vi "differentiator.vi"(10 "X-YCluster":cluster{"Array":dbl[], "Array":dbl[]}) -> (1 "sign":dbl[](array[numeric]), 2 "deltaY/deltaX":dbl[](array[numeric]) format="%#.2f")   [LabVIEW 2022 SP3]
panel:
  out "Ys":dbl[](array[numeric])
  out "Xs":dbl[](array[numeric]) format="%#.2f"
  # "Computes gradient using central difference method; also reports sign of gradient."
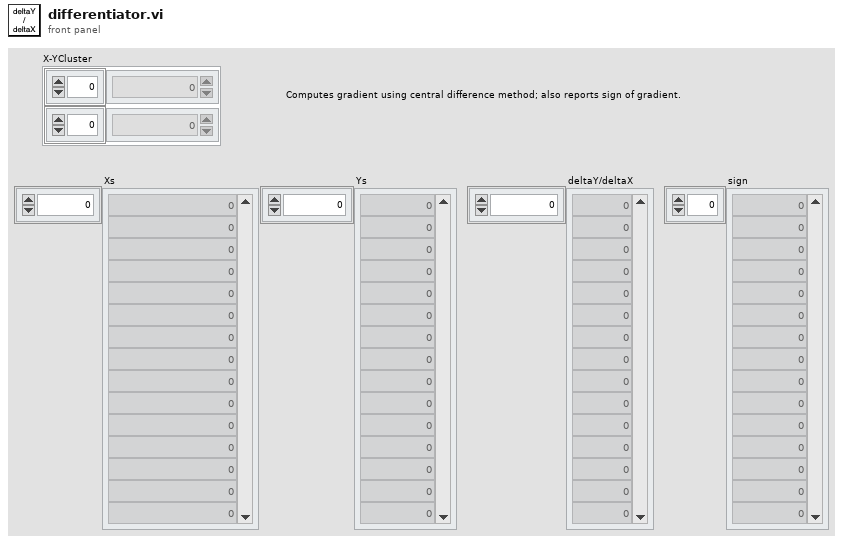
[diagram p1: front panel]
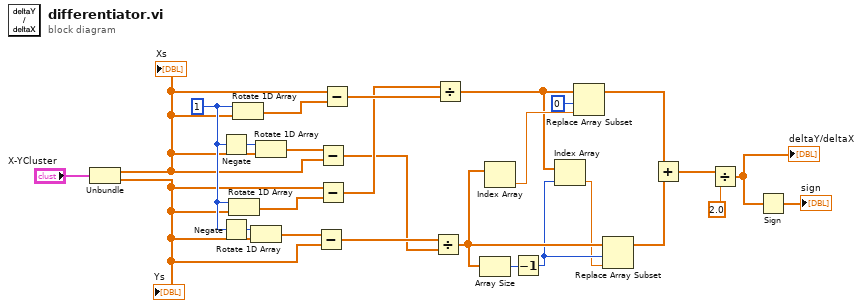
[diagram p0: block diagram]
diagram:
  w20 = 1 ("n")
  n1 = Unbundle("X-YCluster") -> ("Array"=w14:dbl[], "Array"=w17:dbl[])
  "Xs" <- w14
  "Ys" <- w17
  n2 = Negate(x=w20) -> (-x=w19:i32)
  n3 = Negate(x=w20) -> (-x=w21:i32)
  n4 = Rotate 1D Array(1:w17, 2:w20) -> (0:w25:dbl[])
  n5 = Rotate 1D Array(1:w14, 2:w20) -> (0:w26:dbl[])
  n6 = Rotate 1D Array(1:w17, 2:w21) -> (0:w18:dbl[])
  n7 = Rotate 1D Array(1:w14, 2:w19) -> (0:w15:dbl[])
  n8 = Subtract(x=w18, y=w17) -> (x-y=w13:dbl[])
  n9 = Subtract(x=w15, y=w14) -> (x-y=w12:dbl[])
  n10 = Subtract(x=w17, y=w25) -> (x-y=w16:dbl[])
  n11 = Subtract(x=w14, y=w26) -> (x-y=w24:dbl[])
  n12 = Divide(x=w13, y=w12) -> (x/y=w5:dbl[])
  n13 = Divide(x=w16, y=w24) -> (x/y=w3:dbl[])
  n14 = Array Size(array=w5) -> (size(s)=w11:i32)
  n15 = Index Array(array=w5) -> (element=w4:dbl)  [unwired: 1 in]
  n16 = Decrement(x=w11) -> (x-1=w2:i32)
  n17 = Index Array(array=w3, index=w2) -> (element=w1:dbl)
  n18 = Replace Array Subset(array=w3, new element=w4, index=0) -> (w9:dbl[])
  n19 = Replace Array Subset(array=w5, new element=w1, index=w2) -> (w10:dbl[])
  n20 = Add(x=w9, y=w10) -> (x+y=w8:dbl[])
  n21 = Divide(x=w8, y=2.0 ("Numeric")) -> (x/y=w6:dbl[])
  "deltaY/deltaX" <- w6
  n22 = Sign(1:w6) -> (0:→"sign":dbl[])
